vi "Stop Server.vi"(8 "error in":errorcluster, 11 "gRPCid server in":T1) -> (0 "error out":errorcluster)   [LabVIEW 2020, in "grpc-lvsupport-release.lvlib"]
uses:
  gRPC Data Server Engine Windows.llb/grpc-lvsupport-release.lvlib
  gRPC Data Server Engine Windows.llb/grpcId.ctl
  gRPC Data Server Engine Windows.llb/Error Cluster From Error Code.vi
  gRPC Data Server Engine Windows.llb/Simple Error Handler.vi
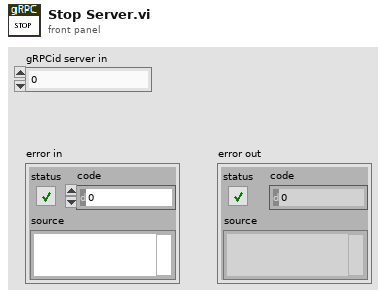
[diagram p1: front panel]
types:
  T1 = typedef "grpc-lvsupport-release.lvlib/grpcId.ctl" = u64
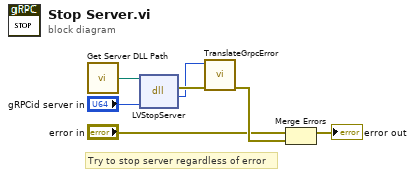
[diagram p0: block diagram]
diagram:
  # "Try to stop server regardless of error"
  n1 = call "Get Server DLL Path.vi"() -> ("Server dll path"=w5:path)
  n2 = dll-call lib="C:/Users/XEnderMD/Desktop/LV gRPC/labview source/gRPC interface/dlls/labview_grpc_server.dll" fn="LVStopServer"(path in=w5, "server"="gRPCid server in") -> (error out=w7:errorcluster, "return type"=w3:i32)  [unwired: 3 in, 1 out]
  n3 = call "TranslateGrpcError.vi"("error in"=w7, "Error Code"=w3) -> ("error out"=w4:errorcluster)  [unwired: 9 in]
  n4 = Merge Errors("error in", w4) -> (→"error out":errorcluster)
